vi "Series from multiple channels.vi"(8 "Row Numbers":i32[](array[numeric]), 9 "Ordinate Index":i32, 10 "Positions In":dbl[](array[numeric]), 11 "Channel Values":string[][](array[string])) -> (0 "Plot?":bool, 1 "Row Numbers Out":i32[](array[numeric]), 2 "Averaged Values":dbl[](array[numeric]), 3 "Positions out":dbl[](array[numeric]), 4 "Plot Metadata":T1)   [LabVIEW 2022 SP3]
uses:
  RFP_Plot_Metadata.ctl
  Error_bars_index.ctl
  <vilib>/Analysis/baseanly.llb/Mean (DBL).vi
  <vilib>/Utility/error.llb/Trim Whitespace One-Sided.vi
  Results_plotter_Global.vi
  <vilib>/Analysis/NI_AALBase.lvlib
  72ef87ad-4fed-40ab-8865-578b4a5455f3.vi
panel:
  out "No of table rows":i32
  out "Number of plot values":i32
  out "Channels":string[](array[string])
  out "element":string
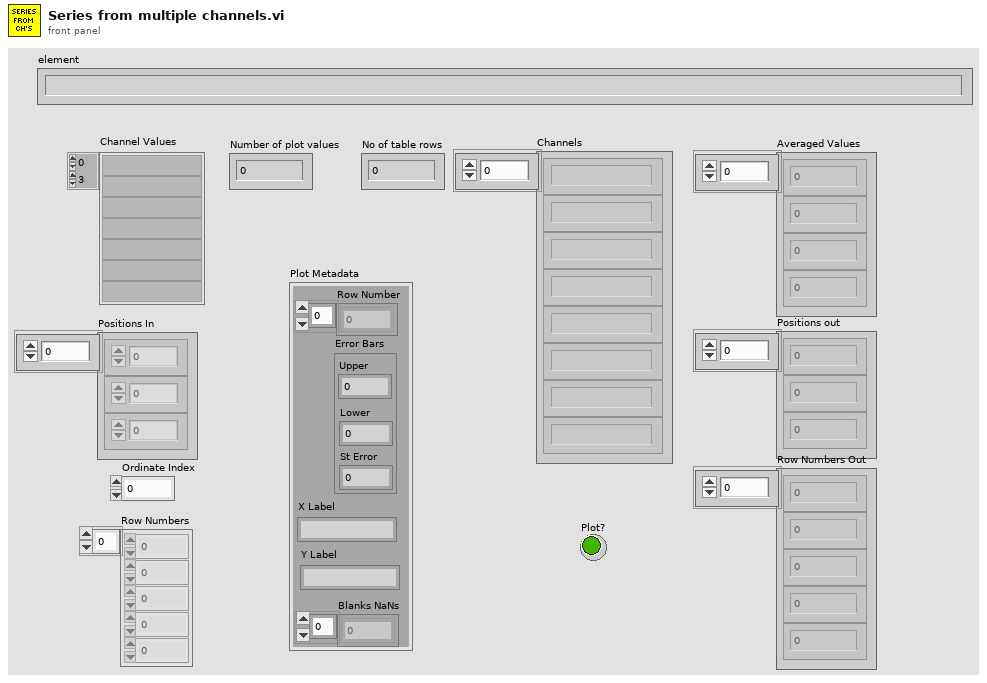
[diagram p1: front panel]
types:
  T1 = typedef "RFP_Plot_Metadata.ctl" = cluster{"Row Number":i32[], "Error Bars":T2, "X Label":string, "Y Label":string, "Blanks NaNs":i32[]}
  T2 = typedef "Error_bars_index.ctl" = cluster{"Upper":i32, "Lower":i32, "St Error":i32}
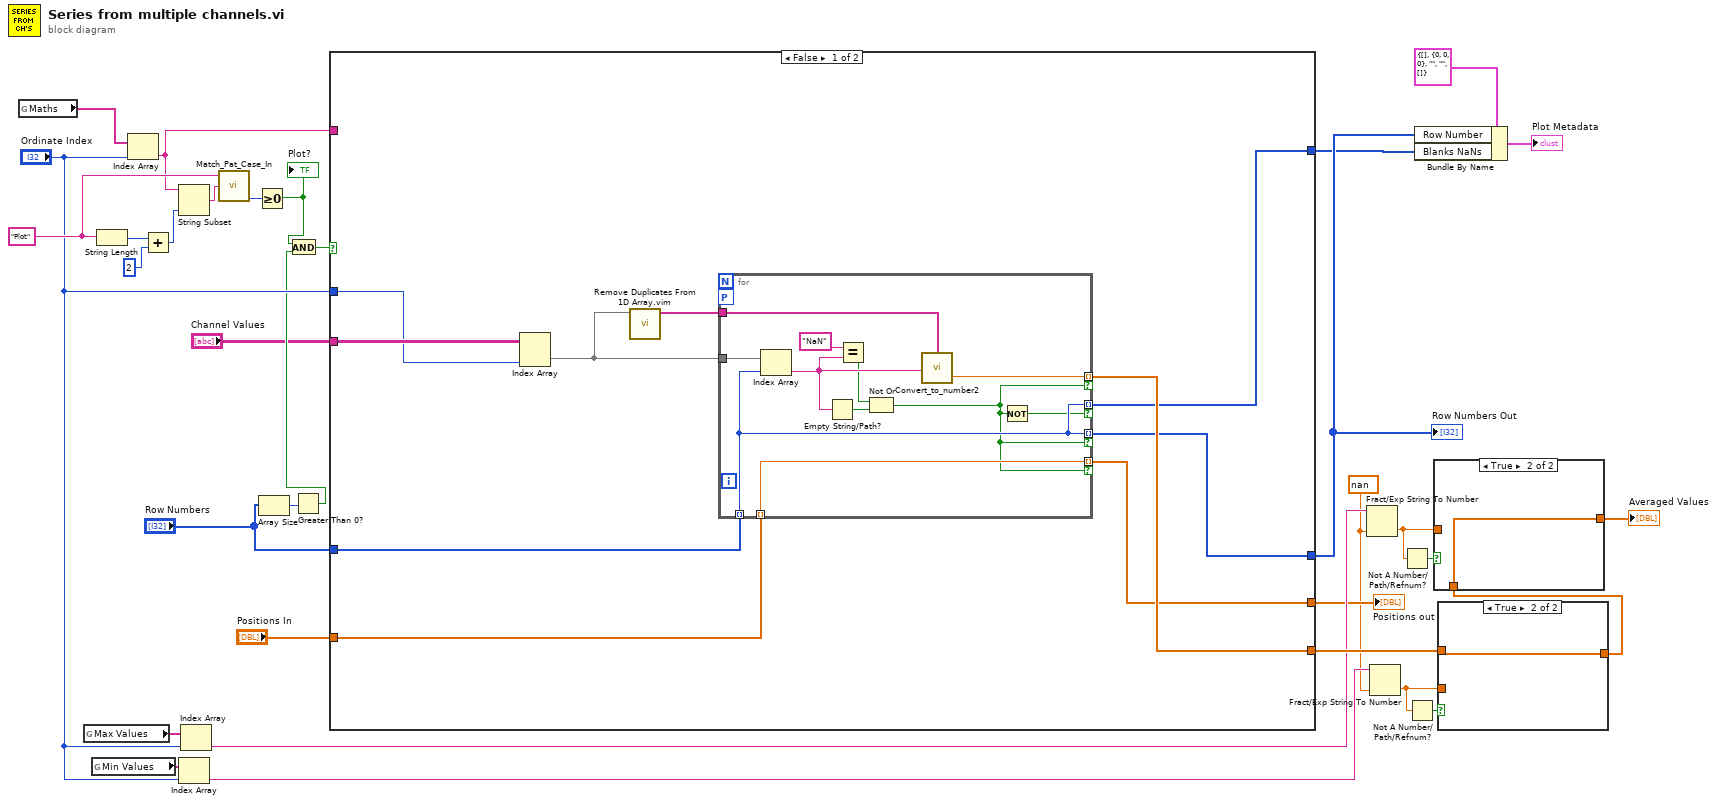
[diagram p0: block diagram]
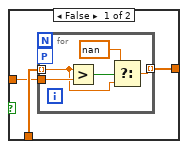
[diagram p2: hidden frame]
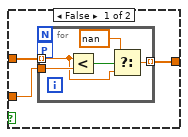
[diagram p3: hidden frame]
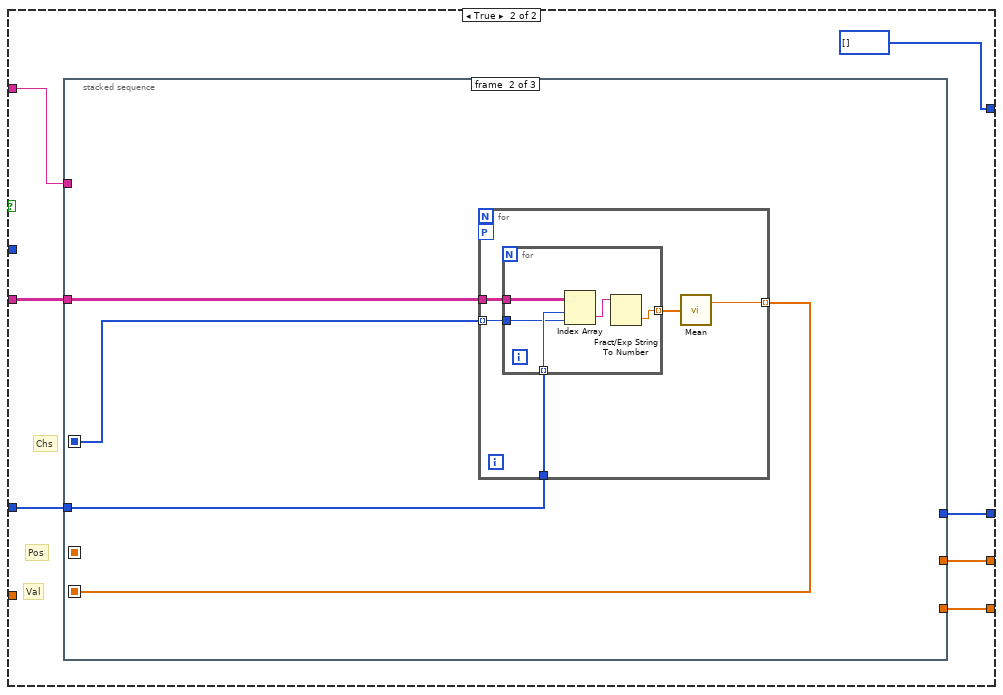
[diagram p4: hidden frame]
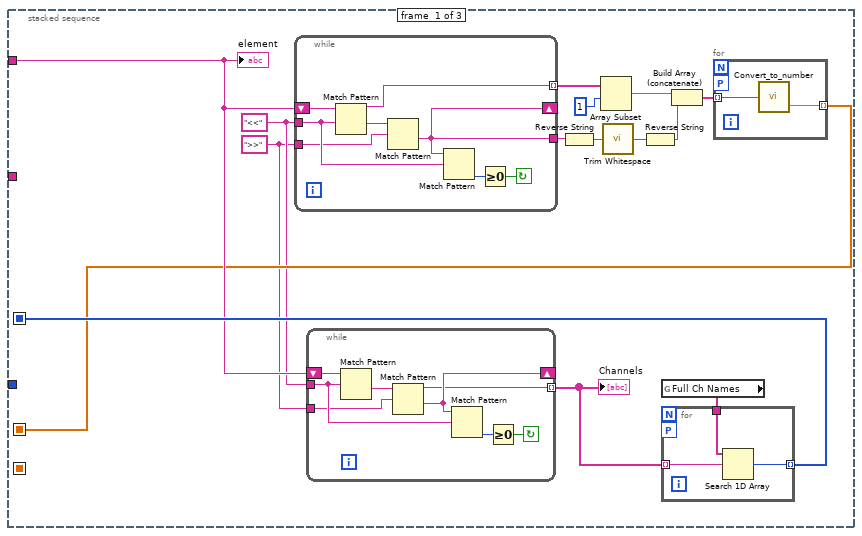
[diagram p5: hidden frame]
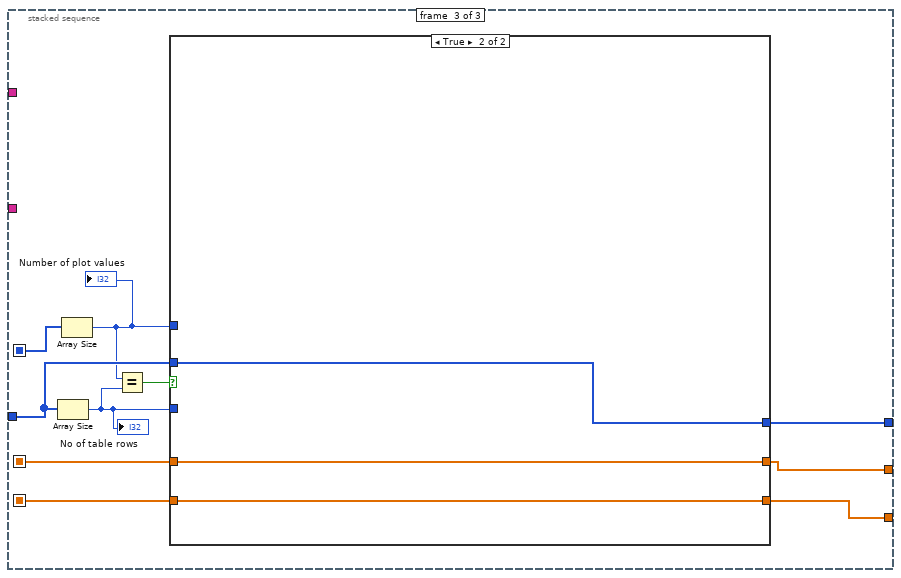
[diagram p6: hidden frame]
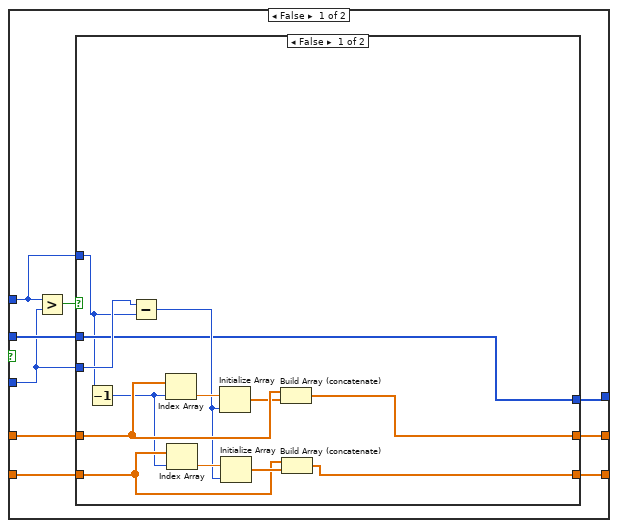
[diagram p7: hidden frame]
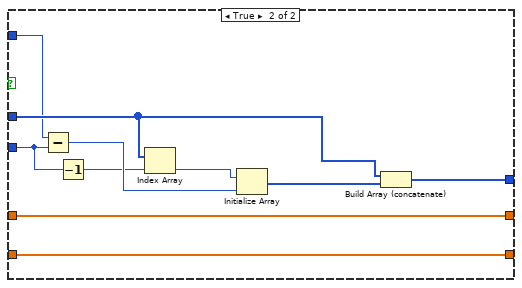
[diagram p8: hidden frame]
diagram:
  w1 = nan ("default (0 DBL)")
  w27 = "Plot" ("regular expression")
  n1 = global read "Results_plotter_Global.vi" "Maths"() -> (w28:string[])
  n2 = global read "Results_plotter_Global.vi" "Max Values"() -> (w24:string[])
  n3 = global read "Results_plotter_Global.vi" "Min Values"() -> (w25:string[])
  n4 = String Length(string=w27) -> (length=w30:i32)
  n5 = Index Array(array=w28, index="Ordinate Index") -> (element=w26:string)
  n6 = Add(x=w30, y=2) -> (x+y=w32:i32)
  n7 = String Subset(string=w26, length (rest)=w32) -> (substring=w33:string)  [unwired: 1 in]
  n8 = Index Array(array=w25, index="Ordinate Index") -> (element=w21:string)
  n9 = Index Array(array=w24, index="Ordinate Index") -> (element=w15:string)
  n10 = call "Match_Pat_Case_In.vi"("String to match"=w27, "String"=w33) -> ("offset past match"=w29:i32)  [unwired: 1 in, 3 out]
  n11 = Greater Or Equal To 0?(x=w29) -> (x >= 0?=w12:bool)
  "Plot?" <- w12
  n12 = Array Size(array="Row Numbers") -> (size(s)=w10:i32)
  n13 = Greater Than 0?(x=w10) -> (x > 0?=w9:bool)
  n14 = And(x=w12, y=w9) -> (x .and. y?=w13:bool)
  n15 = case shown="False" w13 {
    tunnel: "Channel Values" -> [w43 w61]
    tunnel: w26 -> [_ w60]
    tunnel: "Row Numbers" -> [w42 w59]
    tunnel: [w39 w58] -> w3
    tunnel: [w41 w57] -> w22
    tunnel: "Ordinate Index" -> [w40 _]
    tunnel: [w38 w56] -> w8
    tunnel: "Positions In" -> [w37 _]
    tunnel: [w36 i32[] []] -> w2
    frame False {
      n16 = Index Array(array=w43, index (col)=w40) -> (element=w35:string[])  [unwired: 1 in]
      n17 = call "Remove Duplicates From 1D Array.vim"("array"=w35) -> ("array with duplicates removed"=w34:string[])  [unwired: 10 in]
      n18 = for {
        tunnel: w42 -> [w47] mode=indexing
        tunnel: w35 -> [w54]
        tunnel: [w53] -> w41 mode=indexing if=w45
        tunnel: [w47] -> w39 mode=indexing if=w45
        tunnel: [w52] -> w38 mode=indexing if=w45
        tunnel: w37 -> [w52] mode=indexing
        tunnel: [w47] -> w36 mode=indexing if=w46
        workers-P: _ -> [_]
        tunnel: w34 -> [w44]
        n19 = Index Array(array=w54, index=w47) -> (element=w51:string)
        n20 = Empty String/Path?(string/path=w51) -> (empty?=w49:bool)
        n21 = Equal?(x="NaN", y=w51) -> (x = y?=w48:bool)
        n22 = Not Or(1:w49, 2:w48) -> (0:w45:bool)
        n23 = call "Convert_to_number2.vi"("Array - String"=w44, "string"=w51) -> ("Number"=w53:dbl)  [unwired: 2 in, 1 out]
        n24 = Not(x=w45) -> (.not. x?=w46:bool)
      }
    }
    frame True {
      # "Val"
      # "Pos"
      # "Chs"
      n25 = stacked-sequence {
        seq-local: [w67 _ _] -> [_ w100 w121]
        seq-local: [w64 _ _] -> [_ _ w117]
        seq-local: [_ w98 _] -> [_ _ w116]
        tunnel: w61 -> [_ w101 _]
        tunnel: w60 -> [w66 _ _]
        tunnel: w59 -> [_ w99 w118]
        tunnel: [_ _ w119] -> w58
        tunnel: [_ _ w113] -> w57
        tunnel: [_ _ w112] -> w56
        frame #0 {
          w62 = ">>" ("regular expression")
          w63 = "<<" ("regular expression")
          n26 = while {
            shift-left: w66 -> [w97]
            shift-right: [w92] -> _
            tunnel: [w93] -> w70 mode=indexing
            tunnel: [w92] -> w73
            tunnel: w63 -> [w91]
            tunnel: w62 -> [w90]
            stop <- w94 continue-if-true
            n27 = Match Pattern(string=w97, regular expression=w91) -> (before substring=w93:string, after substring=w96:string)  [unwired: 3 out]
            n28 = Match Pattern(string=w96, regular expression=w90) -> (after substring=w92:string)  [unwired: 4 out]
            n29 = Match Pattern(string=w92, regular expression=w91) -> (offset past match=w95:i32)  [unwired: 4 out]
            n30 = Greater Or Equal To 0?(x=w95) -> (x >= 0?=w94:bool)
          }
          n31 = while {
            tunnel: [w84] -> w68 mode=indexing
            shift-left: w66 -> [w89]
            shift-right: [w87] -> _
            tunnel: w63 -> [w83]
            tunnel: w62 -> [w82]
            stop <- w85 continue-if-true
            n32 = Match Pattern(string=w89, regular expression=w83) -> (after substring=w88:string)  [unwired: 4 out]
            n33 = Match Pattern(string=w88, regular expression=w82) -> (before substring=w84:string, after substring=w87:string)  [unwired: 3 out]
            n34 = Match Pattern(string=w87, regular expression=w83) -> (offset past match=w86:i32)  [unwired: 4 out]
            n35 = Greater Or Equal To 0?(x=w86) -> (x >= 0?=w85:bool)
          }
          "Channels" <- w68
          n36 = Reverse String(1:w73) -> (0:w74:string)
          n37 = Array Subset(array=w70, index=1) -> (w71:string[])  [unwired: 1 in]
          n38 = call <vilib>:"Trim Whitespace.vi"("string"=w74) -> ("trimmed string"=w75:string)  [unwired: 1 in]
          n39 = Reverse String(1:w75) -> (0:w76:string)
          n40 = global read "Results_plotter_Global.vi" "Full Ch Names"() -> (w69:string[])
          n41 = for {
            tunnel: w69 -> [w81]
            tunnel: w68 -> [w80] mode=indexing
            tunnel: [w79] -> w67 mode=indexing
            workers-P: _ -> [_]
            n42 = Search 1D Array(1D array=w81, element=w80) -> (index of element=w79:i32)  [unwired: 1 in]
          }
          n43 = Build Array (concatenate)(w71, w76) -> (w65:string[])
          n44 = for {
            tunnel: w65 -> [w78] mode=indexing
            tunnel: [w77] -> w64 mode=indexing
            workers-P: _ -> [_]
            n45 = call "Convert_to_number.vi"("string"=w78) -> ("Number"=w77:dbl)  [unwired: 1 out]
          }
          "element" <- w66
        }
        frame #1 {
          n46 = for {
            tunnel: w101 -> [w106]
            tunnel: w99 -> [w105]
            tunnel: w100 -> [w104] mode=indexing
            tunnel: [w102] -> w98 mode=indexing
            workers-P: _ -> [_]
            n47 = for {
              tunnel: w106 -> [w111]
              tunnel: w105 -> [w110] mode=indexing
              tunnel: w104 -> [w109]
              tunnel: [w107] -> w103 mode=indexing
              n48 = Index Array(array=w111, index (row)=w110, index (col)=w109) -> (element=w108:string)
              n49 = Fract/Exp String To Number(string=w108) -> (number=w107:dbl)  [unwired: 3 in, 1 out]
            }
            n50 = call-poly <vilib>:"Mean.vi"("X"=w103) -> ("mean"=w102:dbl)  [unwired: 1 out]
          }
        }
        frame #2 {
          n51 = Array Size(array=w118) -> (size(s)=w114:i32)
          "No of table rows" <- w114
          n52 = Array Size(array=w121) -> (size(s)=w115:i32)
          "Number of plot values" <- w115
          n53 = Equal?(x=w115, y=w114) -> (x = y?=w120:bool)
          n54 = case shown="True" w120 {
            tunnel: [w124 w156] -> w119
            tunnel: w118 -> [w125 w156]
            tunnel: [w129 w155] -> w112
            tunnel: w117 -> [w128 w155]
            tunnel: [w127 w154] -> w113
            tunnel: w116 -> [w126 w154]
            tunnel: w115 -> [w123 _]
            tunnel: w114 -> [w122 _]
            frame False {
              n55 = Greater?(x=w123, y=w122) -> (0:w130:bool)
              n56 = case shown="False" w130 {
                tunnel: [w141 w153] -> w129
                tunnel: w128 -> [w142 w153]
                tunnel: [w134 w152] -> w127
                tunnel: w126 -> [w135 w152]
                tunnel: w125 -> [w133 w150]
                tunnel: [w133 w151] -> w124
                tunnel: w123 -> [w132 w149]
                tunnel: w122 -> [w143 w146]
                frame False {
                  n57 = Decrement(x=w132) -> (x-1=w131:i32)
                  n58 = Subtract(x=w143, y=w132) -> (x-y=w136:i32)
                  n59 = Index Array(array=w142, index=w131) -> (element=w139:dbl)
                  n60 = Index Array(array=w135, index=w131) -> (element=w138:dbl)
                  n61 = Initialize Array(w139, w136) -> (w140:dbl[])
                  n62 = Initialize Array(w138, w136) -> (w137:dbl[])
                  n63 = Build Array (concatenate)(w142, w140) -> (w141:dbl[])
                  n64 = Build Array (concatenate)(w135, w137) -> (w134:dbl[])
                }
                frame True {
                  n65 = Subtract(x=w149, y=w146) -> (x-y=w145:i32)
                  n66 = Decrement(x=w146) -> (x-1=w144:i32)
                  n67 = Index Array(array=w150, index=w144) -> (element=w148:i32)
                  n68 = Initialize Array(w148, w145) -> (w147:i32[])
                  n69 = Build Array (concatenate)(w150, w147) -> (w151:i32[])
                }
              }
            }
            frame True {
            }
          }
        }
      }
    }
  }
  "Row Numbers Out" <- w3
  "Positions out" <- w8
  n70 = Fract/Exp String To Number(string=w15, default (0 dbl)=w1) -> (number=w18:dbl)  [unwired: 2 in, 1 out]
  n71 = Fract/Exp String To Number(string=w21, default (0 dbl)=w1) -> (number=w19:dbl)  [unwired: 2 in, 1 out]
  n72 = Not A Number/Path/Refnum?(number/path/refnum=w18) -> (NaN/Path/Refnum?=w17:bool)
  n73 = Not A Number/Path/Refnum?(number/path/refnum=w19) -> (NaN/Path/Refnum?=w20:bool)
  n74 = Bundle By Name(cluster=T1 {"Row Number"=[], "Error Bars"={"Upper"=0, "Lower"=0, "St Error"=0}, "X Label"="", "Y Label"="", "Blanks NaNs"=[]} ("Plot Metadata"), "Row Number"=w3, "Blanks NaNs"=w2) -> (→"Plot Metadata":T1)
  n75 = case shown="True" w20 {
    tunnel: w22 -> [w159 w165]
    tunnel: [w158 w165] -> w16
    tunnel: w19 -> [w157 _]
    frame False {
      n76 = for {
        tunnel: w157 -> [w164]
        tunnel: w159 -> [w162] mode=indexing
        tunnel: [w160] -> w158 mode=indexing
        workers-P: _ -> [_]
        n77 = Less?(x=w162, y=w164) -> (x < y?=w163:bool)
        n78 = Select(t=nan, s=w163, f=w162) -> (s? t:f=w160:dbl)
      }
    }
    frame True {
    }
  }
  n79 = case shown="True" w17 {
    tunnel: w16 -> [w168 w174]
    tunnel: [w167 w174] -> w14
    tunnel: w18 -> [w166 _]
    frame False {
      n80 = for {
        tunnel: w166 -> [w173]
        tunnel: w168 -> [w171] mode=indexing
        tunnel: [w169] -> w167 mode=indexing
        workers-P: _ -> [_]
        n81 = Greater?(x=w171, y=w173) -> (0:w172:bool)
        n82 = Select(t=nan, s=w172, f=w171) -> (s? t:f=w169:dbl)
      }
    }
    frame True {
    }
  }
  "Averaged Values" <- w14
